vi "MAG INIT.vi"(8 "error in (no error)":errorcluster, 9 "PSU Status In":T2 {"Trip Current" format="%.3f"; "Trip Field" format="%.4f"; "Voltage" format="%.2f"; "Field Constant" format="%.6f"; "MID Setpoint (T)" format="%.4f"; "MID Setpoint (A)" format="%.3f"; "MAX Setpoint (T)" format="%.4f"; "MAX Setpoint (A)" format="%.3f"; "Heater Voltage" format="%.2f"; "V Limit (V)" format="%.2f"; "Ramp Rate (A/s)" format="%.3f"; "Output (A)" format="%.3f"; "Output (T)" format="%.4f"; "Persistent Current" format="%.3f"; "Persistent Field" format="%.4f"}, 10 "Field and Temp Range":T1={"VISA (Magnet)"="COM4", "Fields(T)"=[], "Temps(K)"=[], "VISA (Temp) "="COM1", "Port number (3364)"=3364}, 11 "Queue in":refnum<queue>) -> (0 "error out":errorcluster, 1 "PSU Status Out":T2 {"Trip Current" format="%.3f"; "Trip Field" format="%.4f"; "Voltage" format="%.2f"; "Field Constant" format="%.6f"; "MID Setpoint (T)" format="%.4f"; "MID Setpoint (A)" format="%.3f"; "MAX Setpoint (T)" format="%.4f"; "MAX Setpoint (A)" format="%.3f"; "Heater Voltage" format="%.2f"; "V Limit (V)" format="%.2f"; "Ramp Rate (A/s)" format="%.3f"; "Output (A)" format="%.3f"; "Output (T)" format="%.4f"; "Persistent Current" format="%.3f"; "Persistent Field" format="%.4f"}, 2 "VISA Resource Name Out":refnum<visa-resource-name>, 3 "Queue out":refnum<queue>)   [LabVIEW 2025]
uses:
  <instrlib>/SMS LabVIEW Drivers/Source Code/Public/PSU Status.ctl
  <instrlib>/SMS LabVIEW Drivers/Source Code/Cryogenic Ltd SMSXXX.lvlib
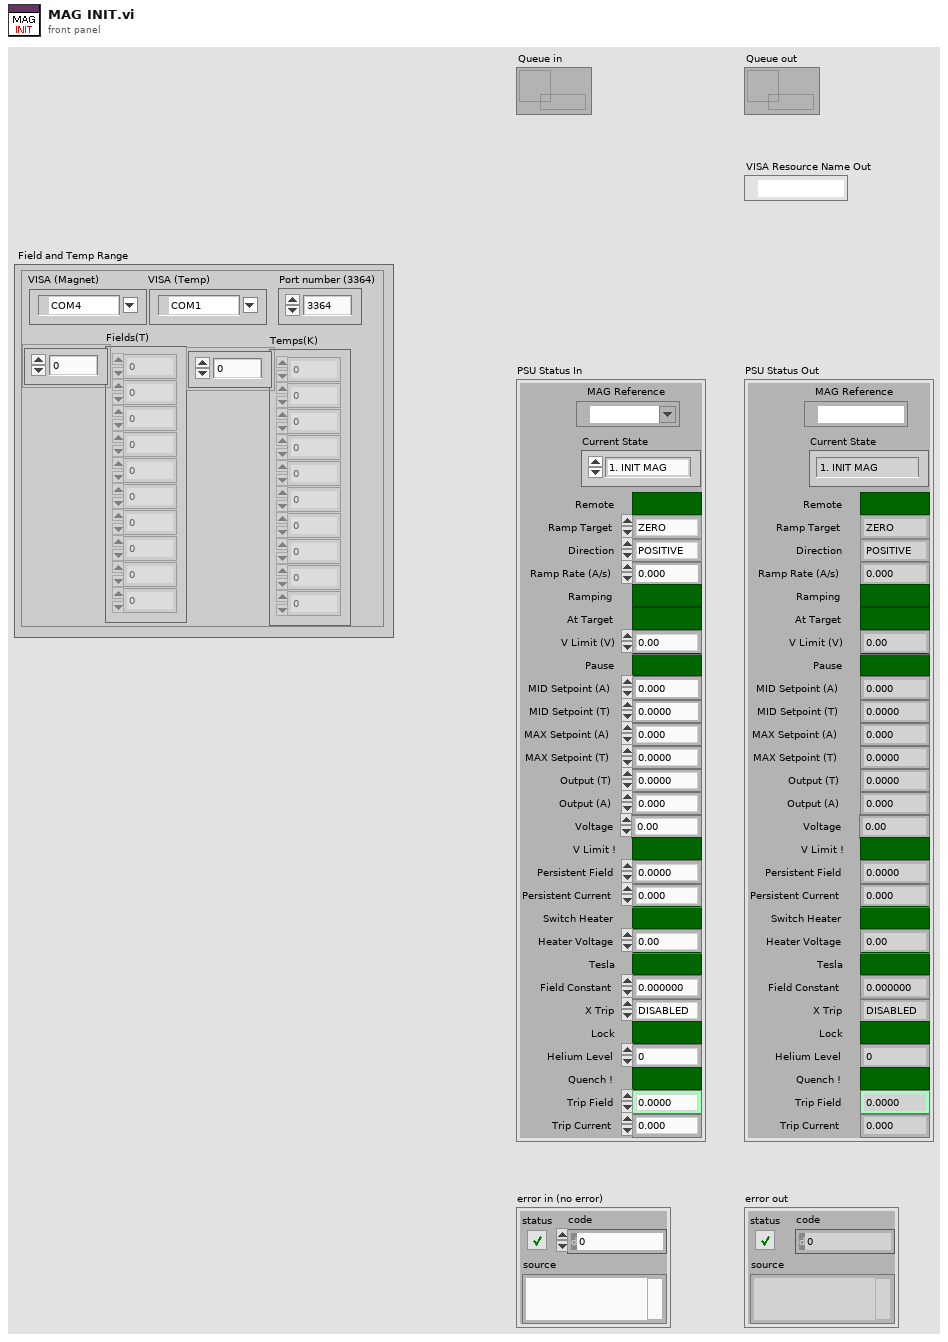
[diagram p1: front panel]
types:
  T1 = cluster{"VISA (Magnet)":refnum<visa-resource-name>, "Fields(T)":dbl[], "Temps(K)":dbl[], "VISA (Temp) ":refnum<visa-resource-name>, "Port number (3364)":u32}
  T2 = typedef "PSU Status.ctl" = cluster{"Ramp Target":enum16{"ZERO", "MID", "MAX"}, "Pause":bool, "Switch Heater":bool, "Persistent Field":dbl, "Persistent Current":dbl, "Tesla":bool, "Output (T)":dbl, "Output (A)":dbl, "X Trip":enum16{"DISABLED", "ENABLED", "ACTIVE"}, "Ramp Rate (A/s)":dbl, "V Limit (V)":dbl, "Heater Voltage":dbl, "MAX Setpoint (A)":dbl, "MAX Setpoint (T)":dbl, "MID Setpoint (A)":dbl, "MID Setpoint (T)":dbl, "Lock":bool, "Field Constant":dbl, "Remote":bool, "Direction":enum16{"POSITIVE", "NEGATIVE", "OPEN", "UNIPOLAR"}, "Helium Level":u16, "Quench !":bool, "Voltage":dbl, "V Limit !":bool, "Ramping":bool, "At Target":bool, "Trip Field":dbl, "Trip Current":dbl, "Current State":enum16{"1. INIT MAG", "2. MAG ON", "3. MAG_STAB", "4. MAG IDLE", "5. PREP NEXT FIELD", "6. APPLY NEXT FIELD", "7. PREP OFF", "8. MAG OFF (Reset)"}, "MAG Reference":refnum<visa-resource-name>}
  T3 = enum16{"1. INIT MAG", "2. MAG ON", "3. MAG_STAB", "4. MAG IDLE", "5. PREP NEXT FIELD", "6. APPLY NEXT FIELD", "7. PREP OFF", "8. MAG OFF (Reset)"}
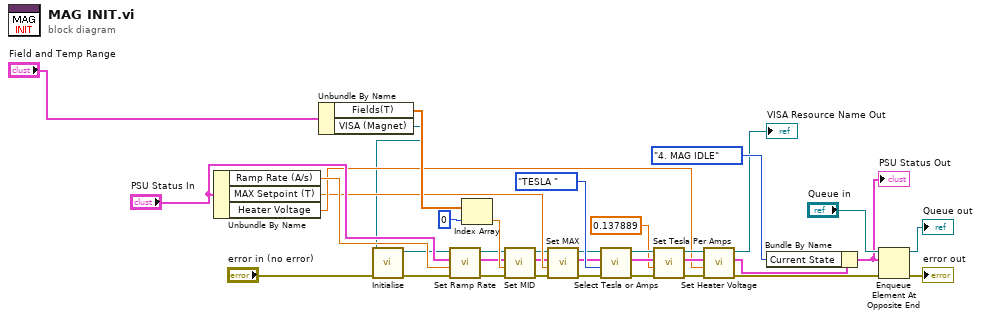
[diagram p0: block diagram]
diagram:
  n1 = Unbundle By Name("PSU Status In") -> ("Ramp Rate (A/s)"=w36:dbl, "MAX Setpoint (T)"=w9:dbl, "Heater Voltage"=w13:dbl)
  n2 = Unbundle By Name("Field and Temp Range") -> ("Fields(T)"=w33:dbl[], "VISA (Magnet)"=w1:refnum<visa-resource-name>)
  n3 = call <instrlib>:"Initialise.vi"("error in"="error in (no error)", "SMS VISA resource name IN"=w1) -> ("error out"=w20:errorcluster, "VISA Resource Name Out"=w19:refnum<visa-resource-name>)  [unwired: 8 in]
  n4 = call <instrlib>:"Set Ramp Rate.vi"("Error in (no error)"=w20, "Ramp Rate (A/s)"=w36, "PSU Status In"="PSU Status In", "VISA Resource Name In"=w19) -> ("Error out"=w8:errorcluster, "PSU Status Out"=w7:T2, "VISA Resource Name Out"=w6:refnum<visa-resource-name>)  [unwired: 4 in, 1 out]
  n5 = Index Array(array=w33, index=0) -> (element=w35:dbl)
  n6 = call <instrlib>:"Set MID.vi"("Error in (no error)"=w8, "MID (T or A)"=w35, "PSU Status In"=w7, "VISA Resource Name In"=w6) -> ("Error out"=w3:errorcluster, "PSU Status Out"=w4:T2, "VISA Resource Name Out"=w5:refnum<visa-resource-name>)  [unwired: 4 in, 1 out]
  n7 = call <instrlib>:"Set MAX.vi"("Error in (no error)"=w3, "MAX  (T or A)"=w9, "PSU Status In"=w4, "VISA Resource Name In"=w5) -> ("Error out"=w23:errorcluster, "PSU Status Out"=w22:T2, "VISA Resource Name Out"=w21:refnum<visa-resource-name>)  [unwired: 4 in, 1 out]
  n8 = call <instrlib>:"Select Tesla or Amps.vi"("Error in (no error)"=w23, "Tesla/Amps"=enum16{"AMPS", "TESLA "}."TESLA ", "PSU Status In"=w22, "VISA Resource Name In"=w21) -> ("Error out"=w24:errorcluster, "PSU Status Out"=w26:T2, "VISA Resource Name Out"=w25:refnum<visa-resource-name>)  [unwired: 4 in, 1 out]
  n9 = call <instrlib>:"Set Tesla Per Amps.vi"("Error in (no error)"=w24, "Tesla Per Amp"=0.137889, "PSU Status In"=w26, "VISA Resource Name In"=w25) -> ("Error out"=w11:errorcluster, "PSU Status Out"=w16:T2, "VISA Resource Name Out"=w28:refnum<visa-resource-name>)  [unwired: 4 in, 1 out]
  n10 = call <instrlib>:"Set Heater Voltage.vi"("Error in (no error)"=w11, "Heater Voltage (V)"=w13, "PSU Status In"=w16, "VISA Resource Name In"=w28) -> ("Error out"=w32:errorcluster, "PSU Status Out"=w17:T2, "VISA Resource Name Out"=→"VISA Resource Name Out":refnum<visa-resource-name>)  [unwired: 4 in, 1 out]
  n11 = Bundle By Name(cluster=w17, "Current State"=T3."4. MAG IDLE") -> (w18:T2)
  "PSU Status Out" <- w18
  n12 = Enqueue Element At Opposite End(queue="Queue in", element=w18, error in (no error)=w32) -> (queue out=→"Queue out":refnum<queue>, error out=→"error out":errorcluster)  [unwired: 1 in, 1 out]
